vi "Write SG Path PM Accessor.vi"(8 "error in (no error)":errorcluster, 10 "STS Scalar Fixture Charact.lvlib:SG Path PM Accessor.lvclass":refnum<class "SG Path PM Accessor Base.lvclass">, 11 "SG Path in":refnum<class "SG Abstract Path.lvclass">) -> (0 "error out":errorcluster, 3 "SG Path out":refnum<class "SG Abstract Path.lvclass">)   [LabVIEW 2023, in "RFFixtureCharact.Public.lvlib" / "SG Abstract Path.lvclass"]
uses:
  SG Abstract Path.lvclass
  Instruments/Power Meter/SG Path PM Accessor Base/SG Path PM Accessor Base.lvclass
  SG Abstract Path.lvclass/SG Abstract Path.ctl
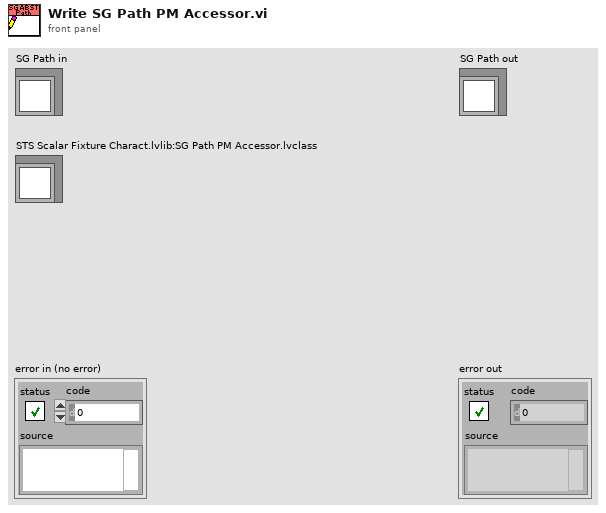
[diagram p1: front panel]
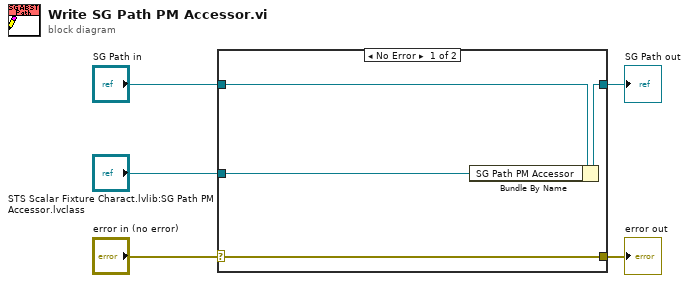
[diagram p0: block diagram]
diagram:
  n1 = case shown="No Error" "error in (no error)" {
    selector: "error in (no error)" -> [w9 w10]
    tunnel: [w9 w10] -> w4
    tunnel: [w7 w11] -> w2
    tunnel: "SG Path in" -> [w8 w11]
    tunnel: "STS Scalar Fixture Charact.lvlib:SG Path PM Accessor.lvclass" -> [w6 _]
    frame No Error {
      n2 = Bundle By Name(cluster=w8, "SG Path PM Accessor"=w6) -> (w7:refnum<class "SG Abstract Path.lvclass">)
    }
    frame Error {
    }
  }
  "error out" <- w4
  "SG Path out" <- w2
